vi "JsonFile Load.vi"(8 "error in (no error)":errorcluster, 11 "Path":path) -> (0 "error out":errorcluster, 3 "Json":string)   [LabVIEW 2019, in "lv-apt-json-file.lvlib"]
uses:
  lv-apt-json-file.lvlib
  <vilib>/Utility/error.llb/Clear Errors.vi
  Json/Remove Comments.vi
  <userlib>/NEVSTOP-Programming-Palette/Configuration/Ini/TextToLines.vi
  <userlib>/_OpenG.lib/array/array.llb/Filter 1D Array__ogtk.vi
  <userlib>/_OpenG.lib/array/array.llb/Filter 1D Array (U8)__ogtk.vi
  <userlib>/NEVSTOP-Programming-Palette/Configuration/Ini/LinesToText.vi
  <vilib>/addons/_JKI.lib/Serialization/JSON/Library/Unflatten From JSON String.vi
  <vilib>/Utility/error.llb/Error Cluster From Error Code.vi
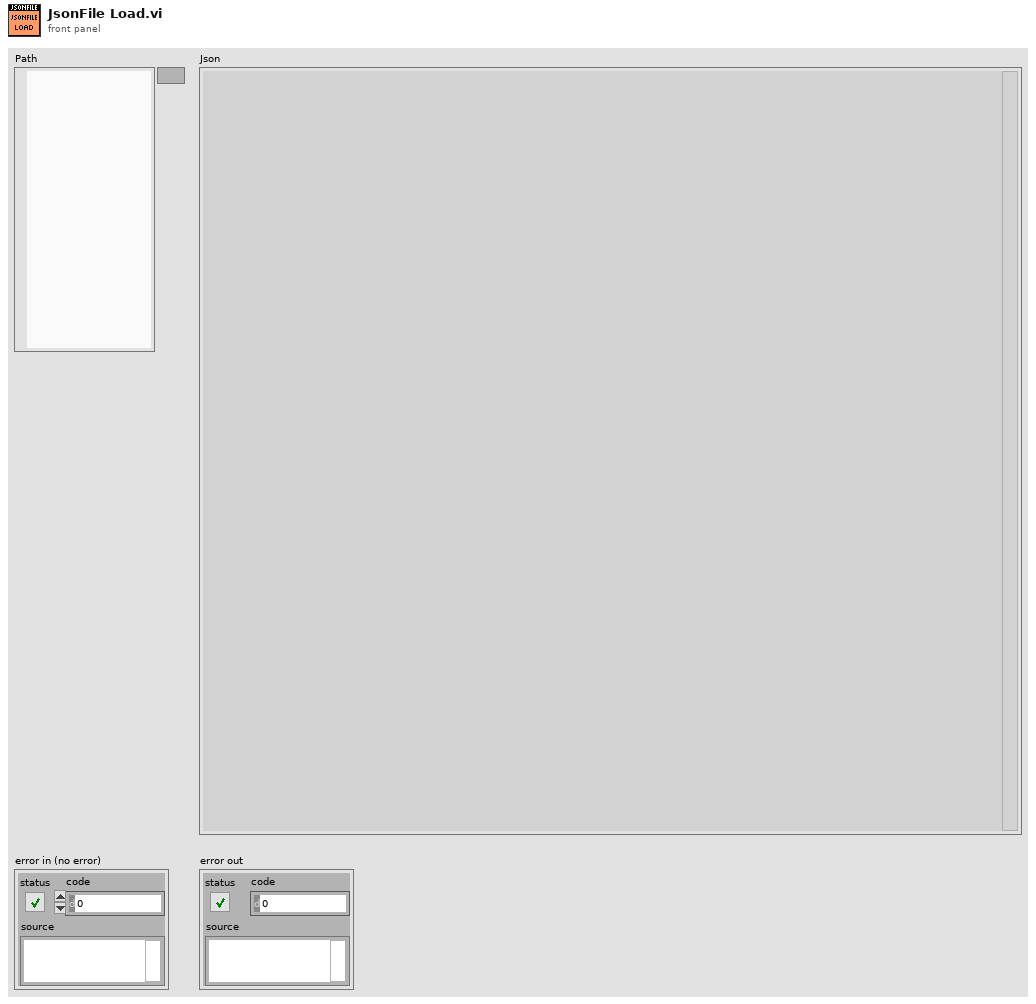
[diagram p1: front panel]
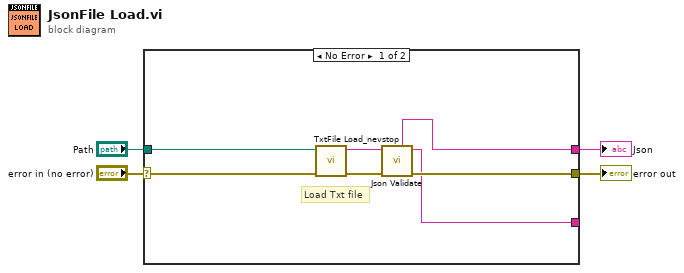
[diagram p0: block diagram]
diagram:
  n1 = case shown="No Error" "error in (no error)" {
    selector: "error in (no error)" -> [w11 w12]
    tunnel: "Path" -> [w10 _]
    tunnel: [w7 _] -> w2
    tunnel: [w8 w12] -> w1
    tunnel: [w5 _] -> _
    frame No Error {
      # "Load Txt file"
      n2 = call <userlib>:"TxtFile Load_nevstop.vi"("error in (no error)"=w11, "Path"=w10) -> ("error out"=w9:errorcluster, "text"=w6:string)  [unwired: 8 in]
      n3 = call "Json Validate.vi"("error in (no error)"=w9, "String"=w6) -> ("error out"=w8:errorcluster, "Json without comments"=w5:string, "String (dup)"=w7:string)  [unwired: 6 in, 1 out]
    }
    frame Error {
    }
  }
  "error out" <- w1
  "Json" <- w2
